vi "Limiter.vi"(8 "error in":errorcluster, 9 "LIMITER_PG_lift-up.LL":dbl, 10 "LIMITER_PG_lift-up.UL in":dbl, 11 "input":dbl) -> (0 "error IO":errorcluster, 1 "low reached":bool, 2 "upper reached":bool, 3 "LIMITER_PG_lift-up.UL out":dbl)   [LabVIEW 2022 SP3]
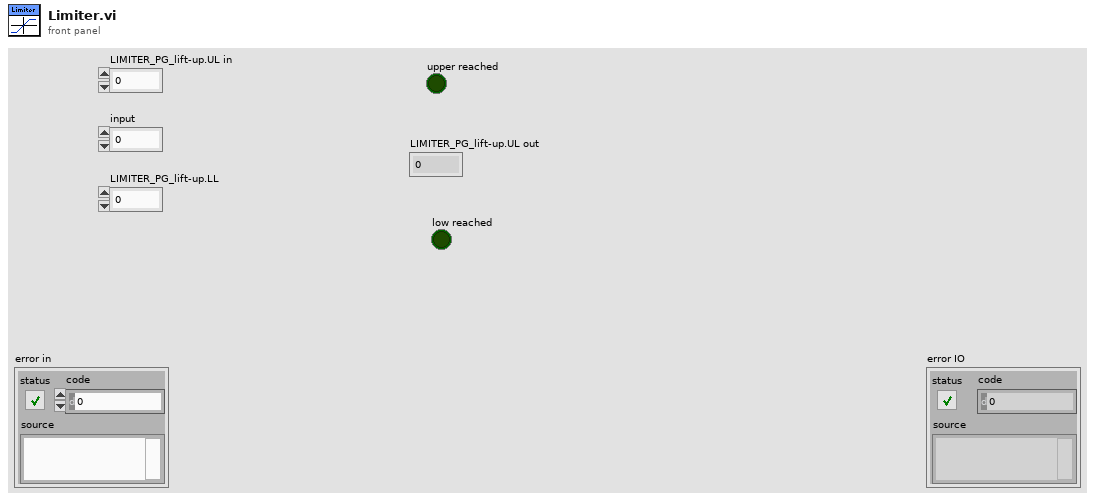
[diagram p1: front panel]
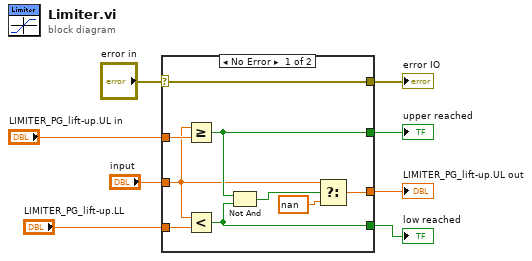
[diagram p0: block diagram]
diagram:
  n1 = case shown="No Error" "error in" {
    selector: "error in" -> [w17 _]
    tunnel: [w17 _] -> w7
    tunnel: "LIMITER_PG_lift-up.UL in" -> [w16 _]
    tunnel: "LIMITER_PG_lift-up.LL" -> [w15 _]
    tunnel: "input" -> [w11 _]
    tunnel: [w14 _] -> w3
    tunnel: [w13 _] -> w2
    tunnel: [w10 _] -> w1
    frame No Error {
      n2 = Greater Or Equal?(x=w11, y=w16) -> (x >= y?=w14:bool)
      n3 = Less?(x=w11, y=w15) -> (x < y?=w13:bool)
      n4 = Not And(1:w13, 2:w14) -> (0:w12:bool)
      n5 = Select(t=w11, s=w12, f=nan) -> (s? t:f=w10:dbl)
    }
    frame Error {
    }
  }
  "error IO" <- w7
  "LIMITER_PG_lift-up.UL out" <- w1
  "upper reached" <- w3
  "low reached" <- w2
